vi "global_parameters_changed.vi"() -> ()   [LabVIEW 2011]
panel:
  out "Parameters changed":bool
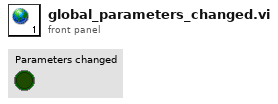
[diagram p1: front panel]
diagram:
